vi "random variable calculate mean.vi"() -> ()   [LabVIEW 2018]
panel:
  out "x/y 2":dbl
  out "x/y":dbl
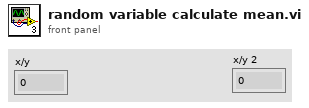
[diagram p1: front panel]
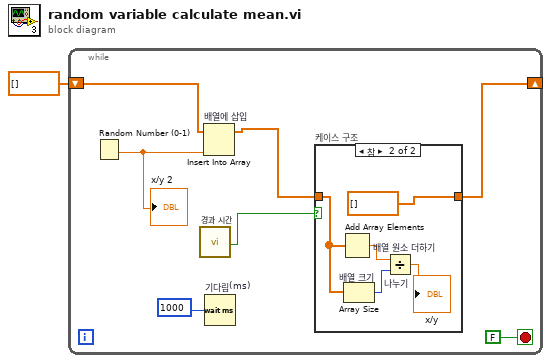
[diagram p0: block diagram]
diagram:
  n1 = while {
    shift-right: [w5] -> _
    shift-left: dbl[] [] -> [w8]
    stop <- FALSE stop-if-true
    n2 = Random Number (0-1)() -> (number: 0 to 1=w2:dbl)
    "x/y 2" <- w2
    n3 = call "경과 시간"() -> ("Time has Elapsed"=w7:bool)  [unwired: 12 in, 7 out]
    n4 = Insert Into Array "배열에 삽입"(array=w8, new element=w2) -> (w6:dbl[])  [unwired: 1 in]
    n5 = Wait (ms) "기다림(ms)"(milliseconds to wait=u32 1000 ("ms 타이머 값")) -> ()  [unwired: 1 out]
    n6 = case "케이스 구조" shown="참" w7 {
      tunnel: [w9 dbl[] []] -> w5
      tunnel: w6 -> [w9 w13]
      frame False {
      }
      frame True {
        n7 = Add Array Elements "배열 원소 더하기"(numeric array=w13) -> (sum=w12:dbl)
        n8 = Array Size "배열 크기"(array=w13) -> (size(s)=w11:i32)
        n9 = Divide "나누기"(x=w12, y=w11) -> (x/y=→"x/y":dbl)
      }
    }
  }
